vi "Close.vi"(8 "error in (no error)":errorcluster, 11 "VISA resource name":refnum<visa-resource-name>) -> (0 "error out":errorcluster)   [LabVIEW 2009, in "JY-SPEX-TRIAX.lvlib"]
doc: "Terminates the software connection to the instrument."
uses:
  JY-SPEX-TRIAX.lvlib
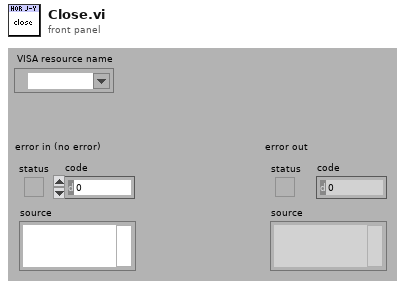
[diagram p1: front panel]
types:
  T1 = typedef "Semaphore RefNum" = refnum<k1>
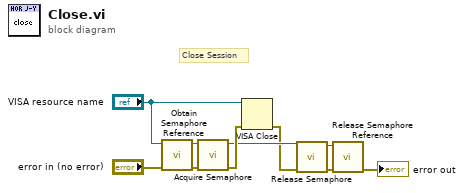
[diagram p0: block diagram]
diagram:
  # "Close Session"
  n1 = call <vilib>:"Obtain Semaphore Reference.vi"("error in (no error)"="error in (no error)", "name (unnamed)"="VISA resource name") -> ("error out"=w10:errorcluster, "semaphore"=w9:T1)  [unwired: 1 in, 3 out]
  n2 = call <vilib>:"Acquire Semaphore.vi"("error in (no error)"=w10, "semaphore"=w9) -> ("error out"=w4:errorcluster, "semaphore out"=w3:T1)  [unwired: 1 in, 3 out]
  n3 = VISA Close(VISA resource name="VISA resource name", error in (no error)=w4) -> (error out=w2:errorcluster)
  n4 = call <vilib>:"Release Semaphore.vi"("error in (no error)"=w2, "semaphore"=w3) -> ("error out"=w8:errorcluster, "semaphore out"=w7:T1)  [unwired: 4 out]
  n5 = call <vilib>:"Release Semaphore Reference.vi"("error in (no error)"=w8, "semaphore"=w7) -> ("error out"=→"error out":errorcluster)  [unwired: 9 out]
